vi "test.vi"() -> ()   [LabVIEW 2024]
panel:
  in  "Vb":i32
  in  "path1 (folder + filename)":string="H:\\My Drive\\Lab\\PPMS\\Measurement\\GaN_1000C_2min_34_56"
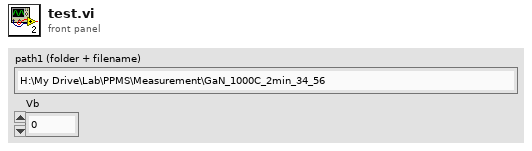
[diagram p1: front panel]
types:
  T1 = enum16{"open", "replace", "create", "open or create", "replace or create", "replace or create with confirmation"}
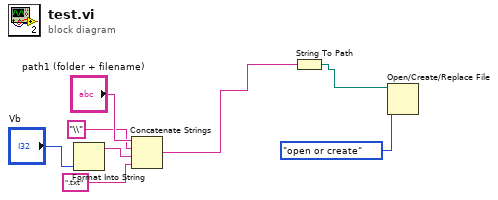
[diagram p0: block diagram]
diagram:
  n1 = Format Into String("Vb") -> (resulting string=w5:string)  [unwired: 3 in, 1 out]
  n2 = Concatenate Strings("path1 (folder + filename)", "\\" ("string"), w5, ".txt" ("string")) -> (w1:string)
  n3 = String To Path(string=w1) -> (path=w2:path)
  n4 = Open/Create/Replace File(file path (use dialog)=w2, operation (0:open)=T1."open or create") -> ()  [unwired: 4 in, 3 out]
